vi "Example MS Chart.vi"() -> ()   [LabVIEW 2015]
uses:
  Controls/Chart.ctl
  Controls/Title.ctl
  Controls/Legend.ctl
  Controls/3D.ctl
  Controls/Series.ctl
  Controls/Marker.ctl
  MSChart/Add Points to Series_DBL[].vi
  MSChart/Add Points to Series_DBL-DBL-Name.vi
  MSChart/Add Points to Series_DBL-DBL[].vi
  MSChart/Add Points to Series_DBL.vi
  System.Windows.Forms.DataVisualization
  Graph Extensions MSChart.lvlib
panel:
  in  "Series":T1[](array[typedef])=[{"ChartType"=13, "Name"="chartName", "Palette"=enum."None", "BorderDashStyle"=enum."Solid", "YAxisType"=enum."Secondary", "XAxisType"=enum."Primary", "BorderColor"=0, "Thickness"=0.0, "Color"=16711717, "Alpha"=192, "Marker"={"MarkerStyle"=enum."Circle", "Size"=12, "Color"=16729410, "Step"=1}}, {"ChartType"=13, "Name"="ItemList", "Palette"=enum."None", "BorderDashStyle"=enum."Solid", "YAxisType"=enum."Secondary", "XAxisType"=enum."Primary", "BorderColor"=0, "Thickness"=0.0, "Color"=2783999, "Alpha"=181, "Marker"={"MarkerStyle"=enum."Triangle", "Size"=12, "Color"=255, "Step"=1}}] {"Alpha" scale=0.0..255.0; "ChartType" items=["Point", "FastPoint", "Bubble", "Line", "Spline", "StepLine", "FastLine", "Bar", "StackedBar", "StackedBar100", "Column", "StackedColumn", "StackedColumn100", "Area", "SplineArea", "StackedArea", "StackedArea100", "Pie", "Doughnut", "Stock", "Candlestick", "Range", "SplineRange", "RangeBar", "RangeColumn", "Radar", "Polar", "ErrorBar", "BoxPlot", "Renko", "ThreeLineBreak", "Kagi", "PointAndFigure", "Funnel", "Pyramid"]}
  in  "3D":T3={"Enable 3D"=FALSE, "LightStyle"=enum."Realistic", "PointGapDepth"=150, "PointDepth"=120, "Perspective"=6, "WallWidth"=0}
  in  "Print":bool
  in  "Data 4":cluster{"X":dbl, "Y":dbl[]}[](array[cluster])=[{"X"=0.0, "Y"=[0.25, 0.35]}, {"X"=1.0, "Y"=[0.75, 0.85]}, {"X"=2.0, "Y"=[1.95, 2.252]}, {"X"=3.0, "Y"=[1.6, 1.85]}, {"X"=4.0, "Y"=[2.5, 2.54]}, {"X"=5.0, "Y"=[1.8, 1.95]}, {"X"=6.0, "Y"=[2.26, 2.6]}]
  in  "Save":bool
  in  "Data input type":enum16{"1", "2", "3", "4"}(ring)
  in  "Data 3":cluster{"X":dbl, "Y":dbl, "Name":string}[](array[cluster])=[{"X"=0.0, "Y"=0.25, "Name"="Item 1"}, {"X"=1.0, "Y"=1.3500000000000003, "Name"="Item 2"}, {"X"=2.0, "Y"=2.95, "Name"="Item 3"}, {"X"=3.0, "Y"=2.0, "Name"="Item 4"}, {"X"=4.0, "Y"=1.7000000000000002, "Name"="Item 5"}, {"X"=5.0, "Y"=2.3, "Name"="Item 6"}, {"X"=6.0, "Y"=1.9000000000000001, "Name"="Item 7"}, {"X"=7.0, "Y"=2.0000000000000004, "Name"="Item 8"}]
  in  "Data 2":cluster{"X":dbl, "Y":dbl}[](array[cluster])=[{"X"=0.0, "Y"=0.25}, {"X"=1.0, "Y"=0.75}, {"X"=2.0, "Y"=1.95}, {"X"=3.0, "Y"=1.6}, {"X"=4.0, "Y"=1.6}, {"X"=5.0, "Y"=2.5}, {"X"=6.0, "Y"=1.8}, {"X"=7.0, "Y"=1.26}]
  in  "Data 1":dbl[](array[numeric])=[0.25, 0.75, 1.95, 1.6, 2.5, 1.8, 1.26]
  in  "Chart Options":T4={"ChartName"="Chart", "BorderDashStyle"=enum."Solid", "Bordercolor"=0, "Title"={"Title"="My TItle", "TitleFontSize"=16.0, "fontName"="Arial", "font Color"=0, "Docking"=enum."Top"}, "Legend"={"Docking"=enum."None", "BorderDashStyle"=enum."Solid", "BGKcolor"=14935011, "BGKalpha"=134, "Title"="", "TitleSeparator"=enum."None"}} {"Legend"."BGKalpha" scale=0.0..255.0; "Title"."TitleFontSize" min=4.0 max=100.0}
  out "error out":errorcluster
  in  "Chart":refnum<k24>(container)
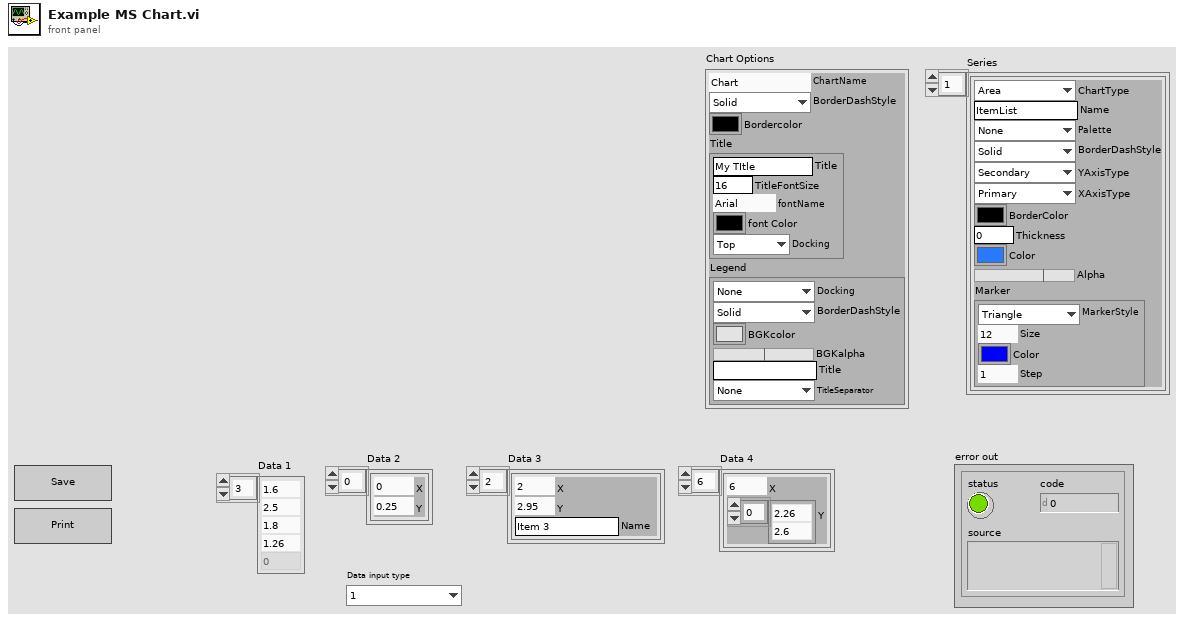
[diagram p1: front panel]
types:
  T1 = typedef "Graph Extensions MSChart.lvlib/Series.ctl" = cluster{"ChartType":i32, "Name":string, "Palette":enum16{"None", "Bright", "Grayscale", "Excel", "Light", "Pastel", "EarthTones", "SemiTransparent", "Berry", "Chocolate", "Fire", "SeaGreen", "BrightPastel"}, "BorderDashStyle":enum16{"NotSet", "Dash", "DashDot", "DashDotDot", "Dot", "Solid"}, "YAxisType":enum16{"Primary", "Secondary"}, "XAxisType":enum16{"Primary", "Secondary"}, "BorderColor":u32, "Thickness":dbl, "Color":u32, "Alpha":u8, "Marker":T2}
  T2 = typedef "Graph Extensions MSChart.lvlib/Marker.ctl" = cluster{"MarkerStyle":enum16{"None", "Square", "Circle", "Diamond", "Triangle", "Cross", "Star4", "Star5", "Star6", "Star10"}, "Size":i32, "Color":u32, "Step":i32}
  T3 = typedef "Graph Extensions MSChart.lvlib/3D.ctl" = cluster{"Enable 3D":bool, "LightStyle":enum16{"None", "Simplistic", "Realistic"}, "PointGapDepth":i32, "PointDepth":i32, "Perspective":i32, "WallWidth":i32}
  T4 = typedef "Graph Extensions MSChart.lvlib/Chart.ctl" = cluster{"ChartName":string, "BorderDashStyle":enum16{"NotSet", "Dash", "DashDot", "DashDotDot", "Dot", "Solid"}, "Bordercolor":u32, "Title":T5, "Legend":T6}
  T5 = typedef "Graph Extensions MSChart.lvlib/Title.ctl" = cluster{"Title":string, "TitleFontSize":dbl, "fontName":string, "font Color":u32, "Docking":enum16{"Top", "Right", "Bottom", "Left"}}
  T6 = typedef "Graph Extensions MSChart.lvlib/Legend.ctl" = cluster{"Docking":enum16{"None", "Top", "Right", "Bottom", "Left"}, "BorderDashStyle":enum16{"NotSet", "Dash", "DashDot", "DashDotDot", "Dot", "Solid"}, "BGKcolor":u32, "BGKalpha":u8, "Title":string, "TitleSeparator":enum16{"None", "Line", "ThickLine", "DoubleLine", "DashLine", "DotLine", "GradientLine", "ThickGradientLine"}}
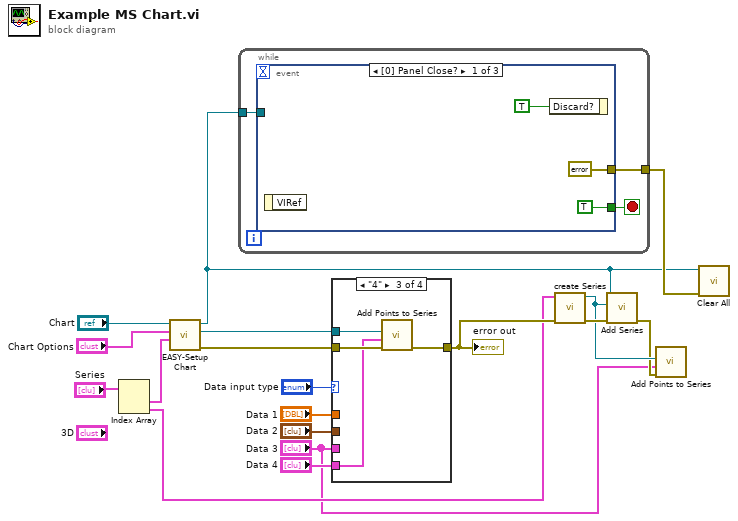
[diagram p0: block diagram]
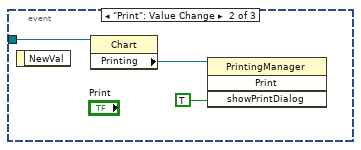
[diagram p2: hidden frame]
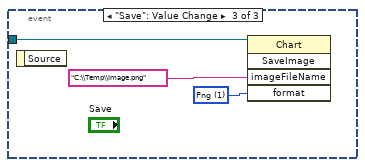
[diagram p3: hidden frame]
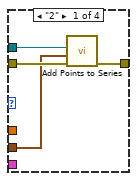
[diagram p4: hidden frame]
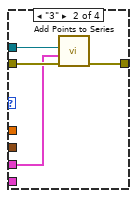
[diagram p5: hidden frame]
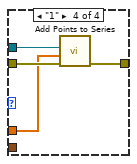
[diagram p6: hidden frame]
diagram:
  n1 = Index Array(array="Series") -> (element #1=w8:T1, element #2=w2:T1)  [unwired: 2 in]
  n2 = call "EASY-Setup Chart.vi"("Series"=w8, "Chart Options"="Chart Options", ".NET MSChart"="Chart") -> ("error out"=w14:errorcluster, ".net MSChart Series"=w12:refnum<k24>, ".NET MSChart"=w4:refnum<k24>)  [unwired: 6 in]
  n3 = while {
    tunnel: w4 -> [w21]
    tunnel: [w19] -> w5
    stop <- w20 stop-if-true
    n4 = event shown="[0] Panel Close?" {
      selector: _ -> [_ _ _]
      dyn-events: _ -> [_ _ _]
      timeout: _ -> [_ _ _]
      tunnel: w21 -> [_ w25 w28]
      tunnel: [TRUE ("Discard?") _ _] -> w20
      tunnel: [errorcluster {"status"=FALSE, "code"=0, "source"=""} ("error out") _ _] -> w19
      event Panel Close? {
        (unwired) TRUE ("Discard?")
        n5 = event-data() -> ()  [unwired: 1 in, 1 out]
        n6 = event-data("Discard?"=TRUE) -> ()  [unwired: 1 in, 1 out]
      }
      event "Print": Value Change {
        n7 = event-data() -> ()  [unwired: 1 in, 1 out]
        n8 = property class="Chart"(reference=w25) -> ("Printing"=w27:refnum<k24>)  [unwired: 1 in, 2 out]
        n9 = invoke class="PrintingManager" method="Print"(reference=w27, "showPrintDialog"=TRUE) -> ()  [unwired: 2 in, 4 out]
      }
      event "Save": Value Change {
        w29 = 1 items=["Jpeg", "Png", "Bmp", "Tiff", "Gif", "Emf", "EmfDual", "EmfPlus"] ("format")
        n10 = event-data() -> ()  [unwired: 1 in, 1 out]
        n11 = invoke class="Chart" method="SaveImage"(reference=w28, "imageFileName"="C:\\Temp\\Image.png", "format"=w29) -> ()  [unwired: 2 in, 5 out]
      }
    }
  }
  n12 = case shown="\"4\"" "Data input type" {
    tunnel: [w33 w37 w41 w45] -> w3
    tunnel: "Data 1" -> [_ _ _ w44]
    tunnel: "Data 3" -> [_ w35 _ _]
    tunnel: "Data 4" -> [_ _ w39 _]
    tunnel: w14 -> [w34 w38 w42 w46]
    tunnel: w12 -> [w32 w36 w40 w43]
    tunnel: "Data 2" -> [w31 _ _ _]
    frame "2" {
      n13 = call-poly "Add Points to Series.vi"("error in (no error)"=w34, "Data"=w31, ".NET MSChart Series"=w32) -> ("error out"=w33:errorcluster)  [unwired: 8 in]
    }
    frame "3" {
      n14 = call-poly "Add Points to Series.vi"("error in (no error)"=w38, "Data"=w35, ".NET MSChart Series"=w36) -> ("error out"=w37:errorcluster)  [unwired: 8 in]
    }
    frame "4" {
      n15 = call-poly "Add Points to Series.vi"("error in (no error)"=w42, "Data"=w39, ".NET MSChart Series"=w40) -> ("error out"=w41:errorcluster)  [unwired: 8 in]
    }
    frame "1" {
      n16 = call-poly "Add Points to Series.vi"("error in (no error)"=w46, "Data"=w44, ".NET MSChart Series"=w43) -> ("error out"=w45:errorcluster)  [unwired: 8 in]
    }
  }
  "error out" <- w3
  n17 = call "create Series.vi"("error in (no error)"=w3, "Series"=w2) -> ("error out"=w10:errorcluster, ".net MSChart Series"=w7:refnum<k24>)  [unwired: 8 in]
  n18 = call "Add Series.vi"("error in (no error)"=w10, ".net MSChart Series"=w7, ".NET MSChart"=w4) -> ("error out"=w6:errorcluster)  [unwired: 8 in]
  n19 = call-poly "Add Points to Series.vi"("error in (no error)"=w6, "Data"="Data 3", ".NET MSChart Series"=w7) -> ()  [unwired: 8 in, 1 out]
  n20 = call "Clear All.vi"("error in (no error)"=w5, ".NET MSChart ref"=w4) -> ()  [unwired: 10 in]
